vi "Butterfly Values to Publishable Names.vi"(1 "Butterfly Numbers":dbl[](array[numeric])) -> (0 "Publishable Names":string[](array[string]))   [LabVIEW 2013]
doc: "This VI converts an array of numbers to strings, and appends the \"PI_\" to the rising numbers and \"RL_\" to the falling numbers according to a general butterfly curve."
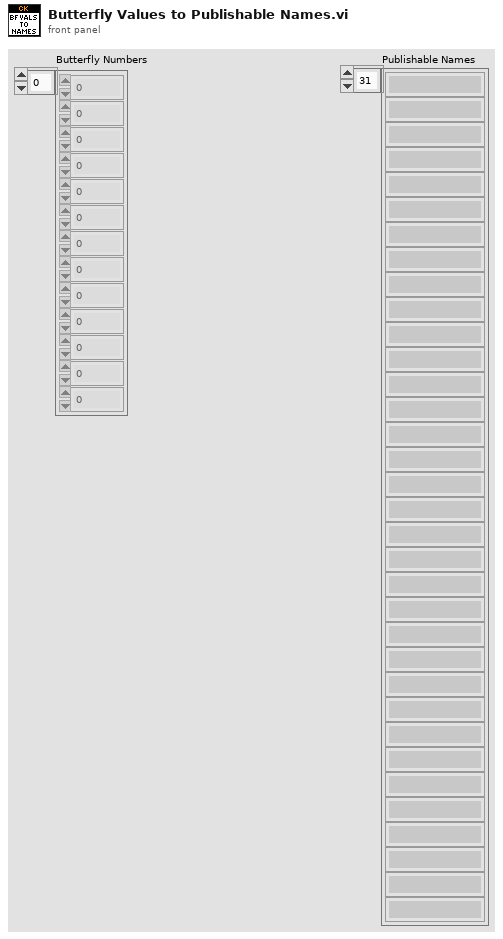
[diagram p1: front panel]
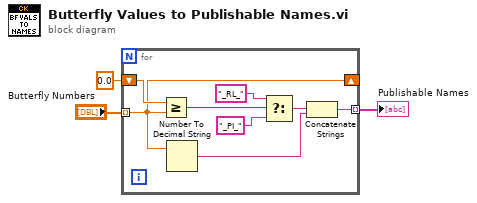
[diagram p0: block diagram]
diagram:
  n1 = for {
    tunnel: "Butterfly Numbers" -> [w7] mode=indexing
    shift-right: [w7] -> _
    shift-left: 0.0 ("Numeric") -> [w11]
    tunnel: [w4] -> w2 mode=indexing
    n2 = Greater Or Equal?(x=w11, y=w7) -> (x >= y?=w10:bool)
    n3 = Number To Decimal String(number=w7) -> (decimal integer string=w5:string)  [unwired: 1 in]
    n4 = Select(t="_RL_", s=w10, f="_PI_") -> (s? t:f=w6:string)
    n5 = Concatenate Strings(w6, w5) -> (w4:string)
  }
  "Publishable Names" <- w2
